vi "EyeTrackingAVI.vi"() -> ()   [LabVIEW 2010]
uses:
  <vilib>/vision/Shape Detection.llb/ShapeDetectionMatchOptions.ctl
  <vilib>/vision/Pattern Matching.llb/IMAQ Match Range Setting.ctl
  <vilib>/vision/Pattern Matching.llb/IMAQ Curve Parameters.ctl
  <instrlib>/niHWS/nihws.llb/niHWS Open File Permissions ID.ctl
  <instrlib>/niHWS/nihws.llb/niHWS Write Analog DBL.vi
  <vilib>/vision/NI_Vision_Development_Module.lvlib
panel:
  in  "Progress":dbl(slide) scale=-1.0..1839.0
  in  "FPS replay":u32=10
  in  "Eye Tolerance":sgl=100.0 format="%.2f"
  in  "Minimum match score":dbl
  out "appended array":cluster{i32, i32}[](array[cluster])
  out "Global Rectangle":i32[](array[numeric])
  out "Points":i32[](array[numeric])
  out "Counter":cluster{"Frame":sgl, "Total ":sgl} {"Total" format="%.2f"; "Frame" format="%.2f"}
  out "Reflection":cluster{"X position":sgl, "Y position":sgl} {"Y position" format="%.2f"; "X position" format="%.2f"}
  in  "Curve Parameters":T1={"Extraction Mode"=0, "Edge Threshold"=90, "Edge Filter Size"=2, "Min Length"=25, "Row Search Step Size"=15, "Col Search Step Size"=15, "Max Endpoint Gap"=10, "Closed"=FALSE, "Subpixel"=FALSE} {"Extraction Mode" items=["Normal", "Uniform Regions"]; "Edge Filter Size" items=["Fine", "Normal", "Contour Tracing"]; "Max Endpoint Gap" min=0; "Col Search Step Size" min=1 max=255 step=1; "Row Search Step Size" min=1 max=255 step=1; "Min Length" min=0; "Edge Threshold" min=1 max=350 step=1}
  in  "Match Options":T2={"Rotation"=TRUE, "Scale"=TRUE, "Occlusion"=FALSE, "Range Settings"=[]} {"Range Settings"."Max" format="%.2f"; "Range Settings"."Min" format="%.2f"; "Range Settings"."Match Constraints" items=["Rotation Angle (degrees)", "Scale Factor (%)", "Occlusion (%)"]}
  in  "Circle Descriptor":cluster{"Min Radius":dbl, "Max Radius":dbl}={"Min Radius"=3.0, "Max Radius"=500.0}
  in  "track":bool
  out "Image":T4(plugin-control)
  in  "Save":bool
  in  "Range":cluster{"Lower value":sgl, "Upper value":sgl}={"Lower value"=0.0, "Upper value"=29.0}
  out "Eye Trace":dbl[][](graph)
  in  "Pupil Color":sgl=150.0
  out "Centroid":cluster{"X Centroid":sgl, "Y Centroid":sgl} {"Y Centroid" format="%.2f"; "X Centroid" format="%.2f"}
  in  "Min Size":dbl=300.0
  in  "Max Size":dbl=25000.0
  in  "AVI Path":path
  in  "stop":bool
  # "Range"
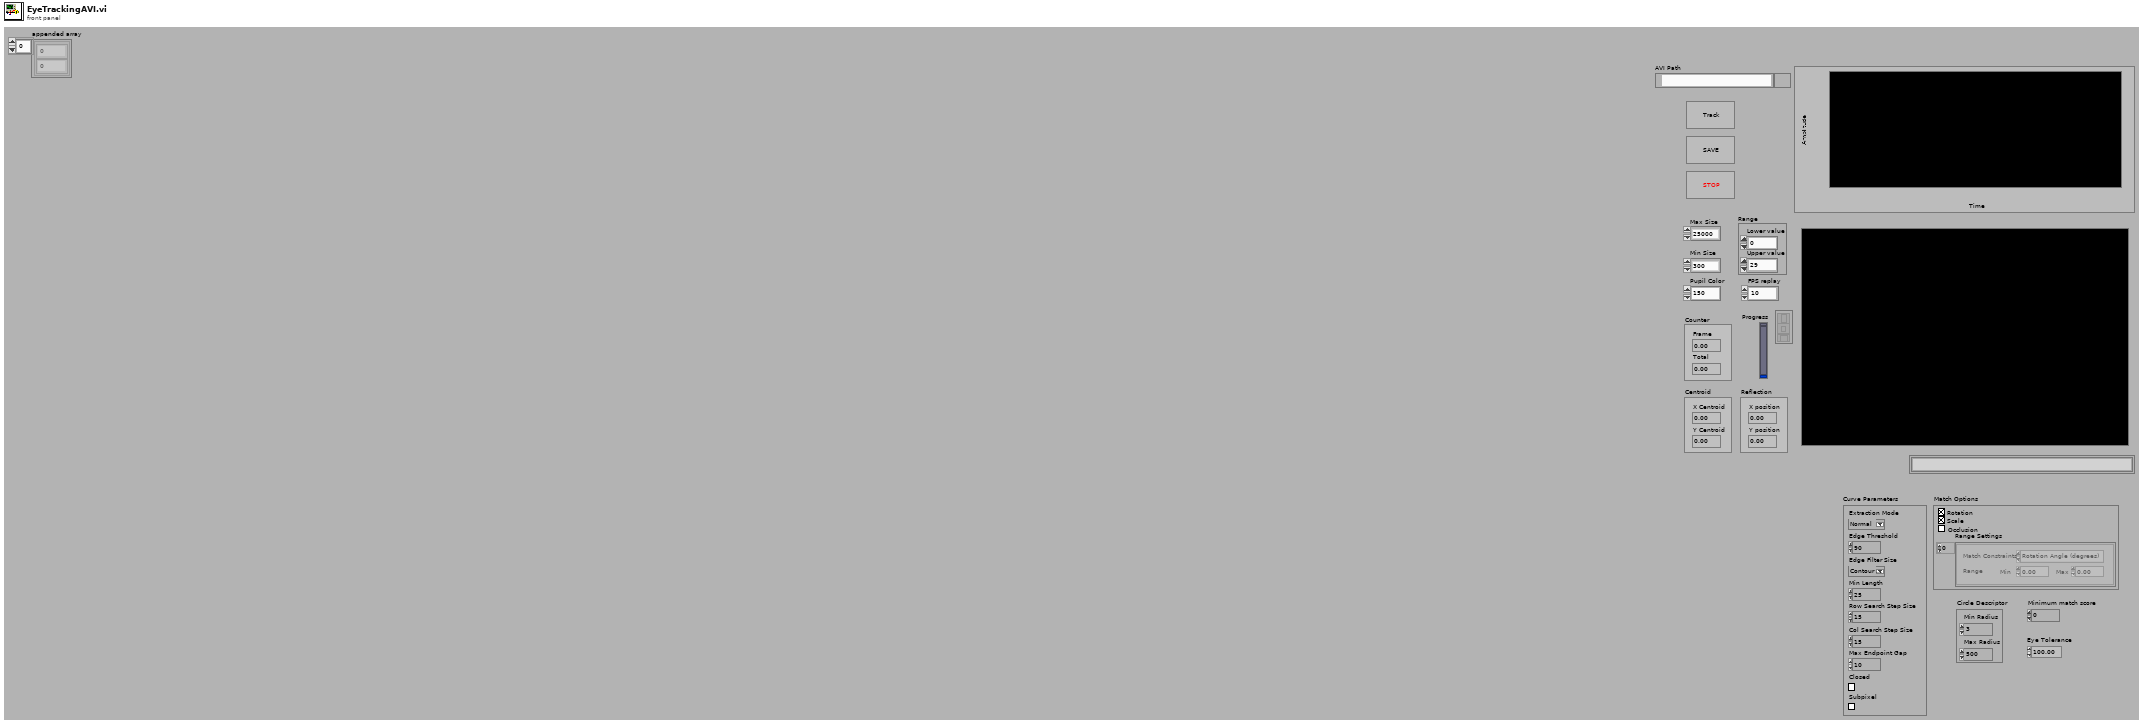
[diagram p1: front panel]
types:
  T1 = typedef "IMAQ Curve Parameters.ctl" = cluster{"Extraction Mode":u32, "Edge Threshold":i32, "Edge Filter Size":u32, "Min Length":i32, "Row Search Step Size":i32, "Col Search Step Size":i32, "Max Endpoint Gap":i32, "Closed":bool, "Subpixel":bool}
  T2 = typedef "ShapeDetectionMatchOptions.ctl" = cluster{"Rotation":bool, "Scale":bool, "Occlusion":bool, "Range Settings":T3[]}
  T3 = typedef "IMAQ Match Range Setting.ctl" = cluster{"Match Constraints":u32, "Min":dbl, "Max":dbl}
  T4 = typedef "IMAQ Image.ctl" = refnum<image>
  T5 = cluster{"Global Rectangle":i32[], "Contours":cluster{"Contour Type":u32, "ROI Type":u32, "Points":i32[]}[]}
  T6 = typedef "IMAQ Circle" = cluster{"Center X":i32, "Center Y":i32, "Inner Radius":i32, "Outer Radius":i32, "Start Angle":dbl, "End Angle":dbl}
  T7 = typedef "niHWS Open File Permissions ID.ctl" = enum32{"Read Only", "Read/Write Existing", "Read/Write/Create New", "Read/Write/Create New Always"}
  T8 = typedef "AviRefnum.ctl" = refnum<k1>
  T9 = cluster{"Contour Type":u32, "ROI Type":u32, "Points":i32[]}[]
  T10 = cluster{"Contour Type":u32, "ROI Type":u32, "Points":i32[]}
  T11 = cluster{"Position":cluster{"X":sgl, "Y":sgl}, "Radius":dbl, "Score":dbl}[]
  T12 = cluster{"Position":cluster{"X":sgl, "Y":sgl}, "Radius":dbl, "Score":dbl}
  T13 = typedef "ROI Descriptor" = cluster{"Global Rectangle":i32[], "Contours":cluster{"ID":enum32{"External", "Internal"}, "Type":u32, "Coordinates":i32[]}[]}
  T14 = cluster{"Global Rectangle":i32[], "Contours":cluster{"Contour Type":u32, "Type":u32, "Coordinates":i32[]}[]}[]
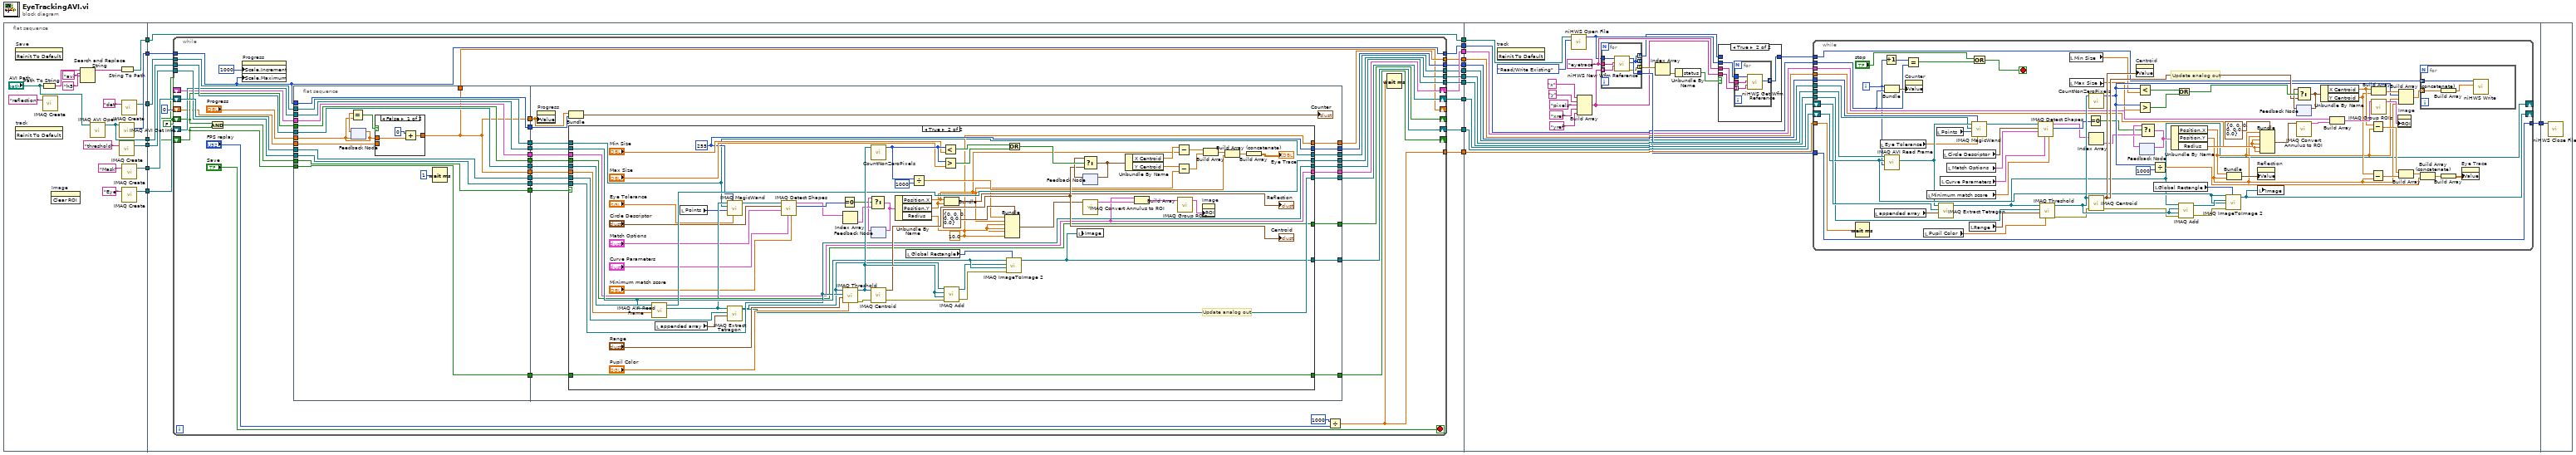
[diagram p0: block diagram]
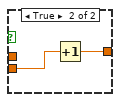
[diagram p2: hidden frame]
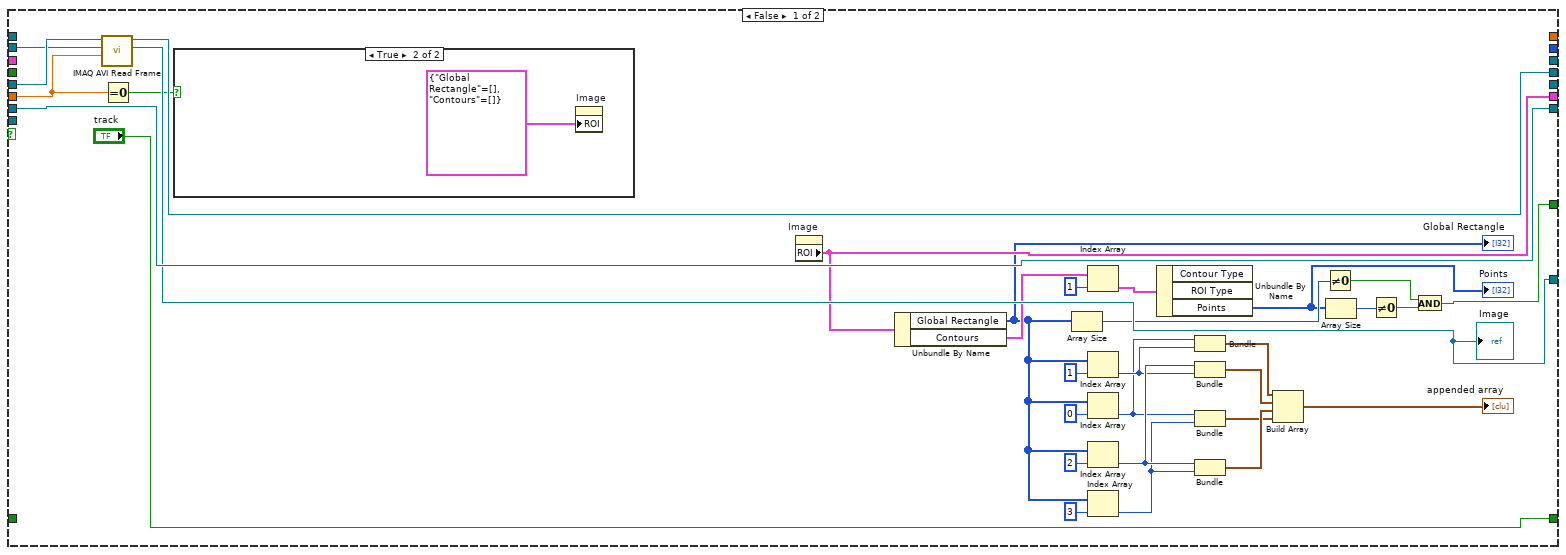
[diagram p3: hidden frame]
diagram:
  n1 = flat-sequence {
    tunnel: [w36] -> w9
    tunnel: [w33] -> w8
    tunnel: [w25] -> w7
    tunnel: [w22] -> w6
    tunnel: [w24] -> w5
    tunnel: [w28] -> w4
    tunnel: [w20] -> w2
    tunnel: [w52] -> w19
    tunnel: [w51] -> w18
    tunnel: [w54] -> w17
    tunnel: [w49] -> w16
    tunnel: [w47] -> w15
    tunnel: [w46] -> w14
    tunnel: [w44] -> w13
    tunnel: [w43] -> w12
    tunnel: [w42] -> w11
    tunnel: [w41] -> w10
    tunnel: w9 -> [w53]
    tunnel: w8 -> [w50]
    tunnel: w7 -> [w55]
    tunnel: w6 -> [w48]
    tunnel: w5 -> [w45]
    tunnel: w4 -> [w43]
    tunnel: w2 -> [w40]
    tunnel: [w39] -> w1
    tunnel: w19 -> [w263]
    tunnel: w18 -> [w262]
    tunnel: w17 -> [w261]
    tunnel: w16 -> [w260]
    tunnel: w15 -> [w259]
    tunnel: w14 -> [w252]
    tunnel: w13 -> [w249]
    tunnel: w12 -> [w248]
    tunnel: w11 -> [w247]
    tunnel: w10 -> [w246]
    tunnel: [w253] -> w3
    tunnel: w1 -> [w245]
    tunnel: w3 -> [w354]
    frame #0 {
      n2 = invoke on="Save" class="Bool (strict)" method="Reinit To Default"() -> ()  [unwired: 3 in, 3 out]
      n3 = invoke on="track" class="Bool (strict)" method="Reinit To Default"() -> ()  [unwired: 3 in, 3 out]
      n4 = Path To String(path="AVI Path") -> (string=w31:string)
      n5 = call "IMAQ Create"("Image Name"="reflection") -> ()  [unwired: 3 in, 3 out]
      n6 = invoke on="Image" class="ImageControl" method="Clear ROI"() -> ()  [unwired: 3 in, 3 out]
      n7 = Search and Replace String(input string=w31, search string="avi" ("regular expression"), replace string="h5" ("replace string (\"\")")) -> (result string=w32:string)  [unwired: 5 in, 3 out]
      n8 = call "IMAQ AVI Open"("AVI Path"="AVI Path") -> ("Avi Refnum"=w25:T8)  [unwired: 9 in, 1 out]
      n9 = String To Path(string=w32) -> (path=w28:path)
      n10 = call "IMAQ AVI Get Info"("Avi Refnum"=w25) -> ("Number of Frames"=w24:u32)  [unwired: 6 in, 4 out]
      n11 = call "IMAQ Create"("Image Name"="threshold") -> ("New Image"=w22:T4)  [unwired: 3 in, 2 out]
      n12 = call "IMAQ Create"("Image Name"="det") -> ("New Image"=w20:T4)  [unwired: 3 in, 2 out]
      n13 = call "IMAQ Create"("Image Name"="Mask") -> ("New Image"=w36:T4)  [unwired: 3 in, 2 out]
      n14 = call "IMAQ Create"("Image Name"="Eye") -> ("New Image"=w33:T4)  [unwired: 3 in, 2 out]
    }
    frame #1 {
      w37 = FALSE
      n15 = while {
        shift-right: [w94] -> w52
        shift-left: w53 -> [w93]
        tunnel: w55 -> [w92]
        tunnel: [w91] -> w54
        shift-right: [w95] -> w51
        shift-left: w50 -> [w89]
        tunnel: [w73] -> w49
        tunnel: w48 -> [w90]
        tunnel: [w88] -> w47
        shift-right: [w86] -> _
        shift-left: w37 -> [w85]
        shift-right: [w84] -> w46
        shift-left: _ -> [w83]
        tunnel: w45 -> [w57]
        tunnel: [w57] -> w44
        tunnel: [w82] -> w42
        tunnel: [w81] -> w41
        tunnel: w40 -> [w80]
        tunnel: [w79] -> w39
        shift-right: [w78] -> _
        shift-left: w37 -> [w76]
        shift-right: [w61] -> _
        shift-left: 0 -> [w60]
        stop <- "Save" stop-if-true
        n16 = And(x=w85, y=w76) -> (x .and. y?=w87:bool)
        n17 = property on="Progress" class="Slide (strict)"("Scale.Increment"=1000, "Scale.Maximum"=w57) -> ()  [unwired: 2 in, 2 out]
        n18 = flat-sequence {
          tunnel: w76 -> [w102]
          tunnel: w80 -> [w103]
          tunnel: w57 -> [w104]
          tunnel: w83 -> [w105]
          tunnel: w85 -> [w106]
          tunnel: w87 -> [w107]
          tunnel: w89 -> [w108]
          tunnel: w90 -> [w109]
          tunnel: w92 -> [w110]
          tunnel: w93 -> [w111]
          tunnel: [w111] -> w72
          tunnel: [w110] -> w71
          tunnel: [w109] -> w70
          tunnel: [w108] -> w69
          tunnel: [w107] -> w68
          tunnel: [w106] -> w67
          tunnel: [w105] -> w66
          tunnel: [w104] -> w65
          tunnel: [w103] -> w64
          tunnel: [w102] -> w63
          tunnel: "Progress" -> [w97]
          tunnel: [w96] -> w62
          tunnel: [w96] -> w61
          tunnel: w60 -> [w98]
          tunnel: [w96] -> w59
          tunnel: [w139] -> w95
          tunnel: [w138] -> w94
          tunnel: [w135] -> w91
          tunnel: [w132] -> w88
          tunnel: [w130] -> w86
          tunnel: [w128] -> w84
          tunnel: [w126] -> w82
          tunnel: [w125] -> w81
          tunnel: [w123] -> w79
          tunnel: [w122] -> w78
          tunnel: w72 -> [w137]
          tunnel: w71 -> [w136]
          tunnel: w70 -> [w134]
          tunnel: w69 -> [w133]
          tunnel: w68 -> [w131]
          tunnel: w67 -> [w129]
          tunnel: w66 -> [w127]
          tunnel: w65 -> [w119]
          tunnel: w64 -> [w124]
          tunnel: w63 -> [w121]
          tunnel: w62 -> [w120]
          tunnel: w59 -> [w117]
          frame #0 {
            n19 = feedback #1(w97) -> (w101:dbl)
            n20 = Equal?(x=w101, y=w97) -> (x = y?=w100:bool)
            n21 = feedback-in #1(w97) -> ()
            n22 = case shown="False" w100 {
              tunnel: [w114 w116] -> w96
              tunnel: w98 -> [_ w115]
              tunnel: w97 -> [w113 _]
              frame False {
                n23 = Add(x=0, y=w113) -> (x+y=w114:dbl)
              }
              frame True {
                n24 = Increment(x=w115) -> (x+1=w116:dbl)
              }
            }
            n25 = Wait (ms)(milliseconds to wait=u32 1) -> ()  [unwired: 1 out]
          }
          frame #1 {
            n26 = property on="Progress" class="Slide (strict)"("Value"=w117) -> ()  [unwired: 2 in, 2 out]
            n27 = Bundle(w117, "Number of Frames"=w119) -> (→"Counter":cluster{dbl, "Number of Frames":u32})  [unwired: 1 in]
            n28 = case shown="True" w131 {
              tunnel: [w168 w200] -> w139
              tunnel: [w169 w211] -> w138
              tunnel: w137 -> [w169 w214]
              tunnel: w136 -> [w171 w222]
              tunnel: [w170 w220] -> w135
              tunnel: w133 -> [w167 w215]
              tunnel: w134 -> [_ w213]
              tunnel: [_ w213] -> w132
              tunnel: [w160 w209] -> w130
              tunnel: w129 -> [_ w209]
              tunnel: [w159 w196] -> w128
              tunnel: w127 -> [_ w196]
              tunnel: [_ w182] -> w126
              tunnel: [_ w181] -> w125
              tunnel: w124 -> [_ w177]
              tunnel: [_ w177] -> w123
              tunnel: ["track" w176] -> w122
              tunnel: w121 -> [_ w176]
              tunnel: w120 -> [w140 w173]
              frame False {
                n29 = call "IMAQ AVI Read Frame"("Frame Number"=w140, "Image"=w167, "Avi Refnum"=w171) -> ("Image Out"=w168:T4, "Avi Refnum (duplicate)"=w170:T8)  [unwired: 5 in, 2 out]
                "Image" <- w168
                n30 = Equal To 0?(x=w140) -> (x = 0?=w141:bool)
                n31 = case shown="True" w141 {
                  frame False {
                  }
                  frame True {
                    n32 = property on="Image" class="ImageControl"("ROI"=T5 {"Global Rectangle"=[], "Contours"=[]}) -> ()  [unwired: 2 in, 2 out]
                  }
                }
                n33 = property on="Image" class="ImageControl"() -> ("ROI"=w159:T5)  [unwired: 2 in, 2 out]
                n34 = Unbundle By Name(w159) -> ("Global Rectangle"=w143:i32[], "Contours"=w166:T9)
                "Global Rectangle" <- w143
                n35 = Array Size(array=w143) -> (size(s)=w164:i32)
                n36 = Index Array(array=w166, index=1) -> (element=w165:T10)
                n37 = Index Array(array=w143, index=1) -> (element=w151:i32)
                n38 = Index Array(array=w143, index=0) -> (element=w150:i32)
                n39 = Index Array(array=w143, index=2) -> (element=w152:i32)
                n40 = Index Array(array=w143, index=3) -> (element=w149:i32)
                n41 = Unbundle By Name(w165) -> ("Points"=w157:i32[])  [unwired: 2 out]
                "Points" <- w157
                n42 = Bundle(w150, w151) -> (w148:cluster{i32, i32})  [unwired: 1 in]
                n43 = Bundle(w152, w151) -> (w147:cluster{i32, i32})  [unwired: 1 in]
                n44 = Bundle(w150, w149) -> (w145:cluster{i32, i32})  [unwired: 1 in]
                n45 = Bundle(w152, w149) -> (w146:cluster{i32, i32})  [unwired: 1 in]
                n46 = Build Array(w148, w147, w146, w145) -> (→"appended array":cluster{i32, i32}[])
                n47 = Not Equal To 0?(x=w164) -> (x != 0?=w163:bool)
                n48 = Array Size(array=w157) -> (size(s)=w161:i32)
                n49 = Not Equal To 0?(x=w161) -> (x != 0?=w162:bool)
                n50 = And(x=w163, y=w162) -> (x .and. y?=w160:bool)
              }
              frame True {
                w181 = 10.0 ("Start Angle")
                w182 = u8 255 ("Fill Value")
                # "Update analog out"
                n51 = call "IMAQ AVI Read Frame"("Frame Number"=w173, "Image"=w215, "Avi Refnum"=w222) -> ("Image Out"=w201:T4, "Avi Refnum (duplicate)"=w220:T8)  [unwired: 5 in, 2 out]
                n52 = local read "appended array"() -> (w178:cluster{i32, i32}[])
                n53 = local read "Points"() -> (w180:i32[])
                n54 = call "IMAQ MagicWand"("Tolerance"="Eye Tolerance", "Fill Value"=w182, "Hot spot (x,y)"=w180, "Image Dst"=w177, "Image Src"=w201) -> ("Image Dst Out"=w210:T4)  [unwired: 5 in, 1 out]
                n55 = call-poly "IMAQ Extract Tetragon"("Tetragon"=w178, "Image Dst"=w214, "Image Src"=w201) -> ("Image Dst Out"=w211:T4)  [unwired: 7 in, 1 out]
                n56 = call-poly "IMAQ Detect Shapes"("Minimum match score"="Minimum match score", "Curve Parameters"="Curve Parameters", "Match Options"="Match Options", "Circle Descriptor"="Circle Descriptor", "Image"=w210) -> ("Number of Matches Returned"=w208:i32, "Circles"=w205:T11)  [unwired: 4 in, 1 out]
                n57 = Equal To 0?(x=w208) -> (x = 0?=w202:bool)
                n58 = Index Array(array=w205) -> (element=w207:T12)  [unwired: 1 in]
                n59 = call "IMAQ Threshold"("Replace Value"="Pupil Color", "Range"="Range", "Image Dst"=w213, "Image Src"=w211) -> ("error out"=w235:errorcluster, "Image Dst Out"=w236:T4)  [unwired: 2 in, 4 out]
                n60 = call "CountNonZeroPixels.vi"("Image"=w236) -> ("NonZeroPixels"=w225:i32)  [unwired: 10 out]
                n61 = feedback #2() -> (w204:T12)  [unwired: 1 in]
                n62 = Select(t=w204, s=w202, f=w207) -> (s? t:f=w206:T12)
                n63 = feedback-in #2(w206) -> ()
                n64 = call "IMAQ Centroid"("error in (no error)"=w235, "Image"=w236) -> ("error out"=w234:errorcluster, "Centroid"=w226:cluster{"X Centroid":sgl, "Y Centroid":sgl})  [unwired: 1 in, 1 out]
                "Centroid" <- w226
                n65 = Unbundle By Name(w206) -> ("Position.X"=w184:sgl, "Position.Y"=w183:sgl, "Radius"=w194:dbl)
                n66 = local read "Global Rectangle"() -> (w179:i32[])
                n67 = Divide(x=w225, y=1000) -> (x/y=w223:dbl)
                n68 = Less?(x=w225, y="Min Size") -> (x < y?=w230:bool)
                n69 = Greater?(x=w225, y="Max Size") -> (0:w229:bool)
                n70 = Bundle("X"=w184, "Y"=w183) -> (→"Reflection":cluster{"X":sgl, "Y":sgl})  [unwired: 1 in]
                n71 = call "IMAQ Add"("Image Src A"=w211, "Image Dst"=w236, "Image Src B"=w236, "error in (no error)"=w234) -> ("Image Dst Out"=w212:T4, "error out"=w221:errorcluster)  [unwired: 1 in, 2 out]
                n72 = Bundle(cluster=T6 {"Center X"=0, "Center Y"=0, "Inner Radius"=0, "Outer Radius"=0, "Start Angle"=0.0, "End Angle"=0.0} ("Annulus"), "Center X"=w184, "Center Y"=w183, "Inner Radius"=w194, "Outer Radius"=w194, "Start Angle"=w181, "End Angle"=w181) -> (w193:T6)
                n73 = call "IMAQ ImageToImage 2"("Offset Left/Top"=w179, "error in (no error)"=w221, "Image Dst"=w215, "Image Src (Small)"=w212, "Image Src (Large)"=w215) -> ("Image Dst Out"=w200:T4)  [unwired: 1 in, 5 out]
                n74 = Or(x=w230, y=w229) -> (x .or. y?=w228:bool)
                n75 = local write "Image"(w200) -> ()
                n76 = feedback #3() -> (w227:cluster{"X Centroid":sgl, "Y Centroid":sgl})  [unwired: 1 out]
                n77 = Select(t=w227, s=w228, f=w226) -> (s? t:f=w203:cluster{"X Centroid":sgl, "Y Centroid":sgl})
                n78 = feedback-in #3(w203) -> ()
                n79 = call "IMAQ Convert Annulus to ROI"("Annulus"=w193) -> ("ROI Descriptor"=w199:T13)  [unwired: 8 in, 1 out]
                n80 = Unbundle By Name(w203) -> ("X Centroid"=w187:sgl, "Y Centroid"=w186:sgl)
                n81 = Build Array(w196, w199) -> (w198:T14)
                n82 = Subtract(x=w187, y=w184) -> (x-y=w189:sgl)
                n83 = Subtract(x=w186, y=w183) -> (x-y=w188:sgl)
                n84 = call "IMAQ Group ROIs"("ROI Descriptors"=w198) -> ("ROI Descriptor out"=w197:T13)  [unwired: 3 in, 1 out]
                n85 = property on="Image" class="ImageControl"("ROI"=w197) -> ()  [unwired: 2 in, 2 out]
                n86 = Build Array(w189, w188) -> (w232:sgl[])
                n87 = Build Array (concatenate)(w232, w223) -> (w231:dbl[])
                n88 = Build Array(w231) -> (→"Eye Trace":dbl[][])
              }
            }
          }
        }
        n89 = Divide(x=1000, y="FPS replay") -> (x/y=w73:dbl)
        n90 = Wait (ms)(milliseconds to wait=w73) -> ()  [unwired: 1 out]
      }
    }
    frame #2 {
      w240 = "eyetrace" ("group name (empty)")
      n91 = invoke on="track" class="Bool (strict)" method="Reinit To Default"() -> ()  [unwired: 3 in, 3 out]
      n92 = call <instrlib>:"niHWS Open File.vi"("permissions (0:read only)"=niHWS_Open_File_Permissions_ID."Read/Write Existing", "file path"=w248) -> ("file handle"=w239:u32)  [unwired: 8 in, 1 out]
      n93 = Build Array("x" ("waveform name (empty)"), "y" ("waveform name (empty)"), "pixels" ("waveform name (empty)"), "xref" ("waveform name (empty)"), "yref" ("waveform name (empty)")) -> (w241:string[])
      n94 = for {
        tunnel: w240 -> [w278]
        tunnel: w239 -> [w275]
        tunnel: [w273] -> _ mode=indexing
        tunnel: w241 -> [w277] mode=indexing
        tunnel: [w276] -> w254
        tunnel: [w274] -> w244 mode=indexing
        tunnel: [w273] -> w238 mode=indexing
        n95 = call <instrlib>:"niHWS New Wfm Reference.vi"("waveform name (empty)"=w277, "group name (empty)"=w278, "file handle in"=w275) -> ("error out"=w274:errorcluster, "waveform reference"=w273:u32, "file handle out"=w276:u32)  [unwired: 6 in]
      }
      n96 = Index Array(array=w244) -> (element=w243:errorcluster)  [unwired: 1 in]
      n97 = Unbundle By Name(w243) -> ("status"=w242:bool)
      n98 = case shown="True" w242 {
        tunnel: w241 -> [_ w268]
        tunnel: w240 -> [_ w267]
        tunnel: w239 -> [_ w266]
        tunnel: w238 -> [w264 _]
        tunnel: [w264 w265] -> w237
        frame False {
        }
        frame True {
          n99 = for {
            tunnel: w268 -> [w272] mode=indexing
            tunnel: w267 -> [w271]
            tunnel: w266 -> [w270]
            tunnel: [w269] -> w265 mode=indexing
            n100 = call <instrlib>:"niHWS Get Wfm Reference.vi"("waveform name (empty)"=w272, "group name (empty)"=w271, "file handle in"=w270) -> ("waveform reference"=w269:u32)  [unwired: 6 in, 2 out]
          }
        }
      }
      n101 = while {
        shift-right: [w334] -> _
        shift-left: w262 -> [w335]
        shift-right: [w287] -> _
        shift-left: w263 -> [w336]
        tunnel: w261 -> [w340]
        tunnel: w260 -> [w333]
        tunnel: w259 -> [w322]
        tunnel: w237 -> [w331]
        tunnel: w254 -> [w329]
        tunnel: [w329] -> w253
        tunnel: w252 -> [w310]
        tunnel: w249 -> [w297]
        tunnel: w247 -> [w296]
        tunnel: w246 -> [w295]
        tunnel: w245 -> [w283]
        i -> [w280]
        stop <- w326 stop-if-true
        # "Update analog out"
        n102 = Wait (ms)(milliseconds to wait=w333) -> ()  [unwired: 1 out]
        n103 = local read "appended array"() -> (w284:cluster{i32, i32}[])
        n104 = local read "Eye Tolerance"() -> (w281:sgl)
        n105 = Increment(x=w280) -> (x+1=w279:i32)
        n106 = Bundle(w280, "Number of Frames"=w297) -> (w298:cluster{i32, "Number of Frames":u32})  [unwired: 1 in]
        n107 = call "IMAQ AVI Read Frame"("Frame Number"=w280, "Image"=w335, "Avi Refnum"=w340) -> ("Image Out"=w311:T4)  [unwired: 5 in, 3 out]
        n108 = property on="Counter" class="Clust (strict)"("Value"=w298) -> ()  [unwired: 2 in, 2 out]
        n109 = Equal?(x=w279, y=w297) -> (x = y?=w328:bool)
        n110 = local read "Pupil Color"() -> (w290:sgl)
        n111 = local read "Minimum match score"() -> (w282:dbl)
        n112 = local read "Points"() -> (w286:i32[])
        n113 = call-poly "IMAQ Extract Tetragon"("Tetragon"=w284, "Image Dst"=w336, "Image Src"=w311) -> ("Image Dst Out"=w287:T4)  [unwired: 7 in, 1 out]
        n114 = local read "Curve Parameters"() -> (w291:T1)
        n115 = local read "Circle Descriptor"() -> (w293:cluster{"Min Radius":dbl, "Max Radius":dbl})
        n116 = local read "Match Options"() -> (w292:T2)
        n117 = local read "Range"() -> (w294:cluster{"Lower value":sgl, "Upper value":sgl})
        n118 = call "IMAQ MagicWand"("Tolerance"=w281, "Fill Value"=w296, "Hot spot (x,y)"=w286, "Image Dst"=w283, "Image Src"=w311) -> ("Image Dst Out"=w321:T4)  [unwired: 5 in, 1 out]
        n119 = Or(x="stop", y=w328) -> (x .or. y?=w326:bool)
        n120 = call-poly "IMAQ Detect Shapes"("Minimum match score"=w282, "Curve Parameters"=w291, "Match Options"=w292, "Circle Descriptor"=w293, "Image"=w321) -> ("Number of Matches Returned"=w320:i32, "Circles"=w317:T11)  [unwired: 4 in, 1 out]
        n121 = call "IMAQ Threshold"("Replace Value"=w290, "Range"=w294, "Image Dst"=w322, "Image Src"=w287) -> ("error out"=w349:errorcluster, "Image Dst Out"=w350:T4)  [unwired: 2 in, 4 out]
        n122 = local read "Min Size"() -> (w289:dbl)
        n123 = local read "Max Size"() -> (w288:dbl)
        n124 = Equal To 0?(x=w320) -> (x = 0?=w315:bool)
        n125 = call "CountNonZeroPixels.vi"("Image"=w350) -> ("NonZeroPixels"=w324:i32)  [unwired: 10 out]
        n126 = Index Array(array=w317) -> (element=w319:T12)  [unwired: 1 in]
        n127 = call "IMAQ Centroid"("error in (no error)"=w349, "Image"=w350) -> ("error out"=w348:errorcluster, "Centroid"=w337:cluster{"X Centroid":sgl, "Y Centroid":sgl})  [unwired: 1 in, 1 out]
        n128 = property on="Centroid" class="Clust (strict)"("Value"=w337) -> ()  [unwired: 2 in, 2 out]
        n129 = Less?(x=w324, y=w289) -> (x < y?=w347:bool)
        n130 = Greater?(x=w324, y=w288) -> (0:w346:bool)
        n131 = feedback #4() -> (w316:T12)  [unwired: 1 in]
        n132 = Select(t=w316, s=w315, f=w319) -> (s? t:f=w318:T12)
        n133 = feedback-in #4(w318) -> ()
        n134 = Divide(x=w324, y=1000) -> (x/y=w341:dbl)
        n135 = local read "Global Rectangle"() -> (w285:i32[])
        n136 = Unbundle By Name(w318) -> ("Position.X"=w300:sgl, "Position.Y"=w299:sgl, "Radius"=w313:dbl)
        n137 = Or(x=w347, y=w346) -> (x .or. y?=w345:bool)
        n138 = call "IMAQ Add"("Image Src A"=w287, "Image Dst"=w350, "Image Src B"=w350, "error in (no error)"=w348) -> ("Image Dst Out"=w338:T4, "error out"=w339:errorcluster)  [unwired: 1 in, 2 out]
        n139 = call "IMAQ ImageToImage 2"("Offset Left/Top"=w285, "error in (no error)"=w339, "Image Dst"=w335, "Image Src (Small)"=w338, "Image Src (Large)"=w335) -> ("Image Dst Out"=w334:T4)  [unwired: 1 in, 5 out]
        n140 = Bundle("X"=w300, "Y"=w299) -> (w301:cluster{"X":sgl, "Y":sgl})  [unwired: 1 in]
        n141 = property on="Reflection" class="Clust (strict)"("Value"=w301) -> ()  [unwired: 2 in, 2 out]
        n142 = local write "Image"(w334) -> ()
        n143 = Bundle(cluster=T6 {"Center X"=0, "Center Y"=0, "Inner Radius"=0, "Outer Radius"=0, "Start Angle"=0.0, "End Angle"=0.0} ("Annulus"), "Center X"=w300, "Center Y"=w299, "Inner Radius"=w313, "Outer Radius"=w313, "Start Angle"=w295, "End Angle"=w295) -> (w312:T6)
        n144 = feedback #5() -> (w344:cluster{"X Centroid":sgl, "Y Centroid":sgl})  [unwired: 1 out]
        n145 = Select(t=w344, s=w345, f=w337) -> (s? t:f=w343:cluster{"X Centroid":sgl, "Y Centroid":sgl})
        n146 = feedback-in #5(w343) -> ()
        n147 = call "IMAQ Convert Annulus to ROI"("Annulus"=w312) -> ("ROI Descriptor"=w308:T13)  [unwired: 8 in, 1 out]
        n148 = Unbundle By Name(w343) -> ("X Centroid"=w306:sgl, "Y Centroid"=w304:sgl)
        n149 = Build Array(w310, w308) -> (w309:T14)
        n150 = Subtract(x=w306, y=w300) -> (x-y=w305:sgl)
        n151 = Subtract(x=w304, y=w299) -> (x-y=w303:sgl)
        n152 = Build Array(w306, w304) -> (w325:sgl[])
        n153 = call "IMAQ Group ROIs"("ROI Descriptors"=w309) -> ("ROI Descriptor out"=w307:T13)  [unwired: 3 in, 1 out]
        n154 = property on="Image" class="ImageControl"("ROI"=w307) -> ()  [unwired: 2 in, 2 out]
        n155 = Build Array (concatenate)(w325, w324, w300, w299) -> (w323:sgl[])
        n156 = Build Array(w305, w303) -> (w302:sgl[])
        n157 = for {
          tunnel: w323 -> [w352] mode=indexing
          tunnel: w331 -> [w353] mode=indexing
          n158 = Build Array(w352) -> (w351:sgl[])
          n159 = call-poly <instrlib>:"niHWS Write.vi"("data"=w351, "waveform reference in"=w353) -> ()  [unwired: 8 in, 2 out]
        }
        n160 = Build Array (concatenate)(w302, w341) -> (w330:dbl[])
        n161 = Build Array(w330) -> (w332:dbl[][])
        n162 = property on="Eye Trace" class="WFChart (strict)"("Value"=w332) -> ()  [unwired: 2 in, 2 out]
      }
    }
    frame #3 {
      n163 = call <instrlib>:"niHWS Close File.vi"("file handle"=w354) -> ()  [unwired: 10 in, 1 out]
    }
  }
